vi "Connect To Replacement Terminal.vi"(6 "replacement class term":refnum<vi>, 9 "endpt subvi":refnum<vi>) -> ()   [LabVIEW 2020, in "NI_TargetHelper.lvlib"]
uses:
  <vilib>/TargetSupport/NI_TargetHelper/NI_TargetHelper.lvlib
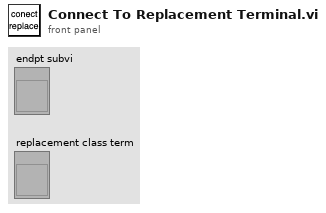
[diagram p1: front panel]
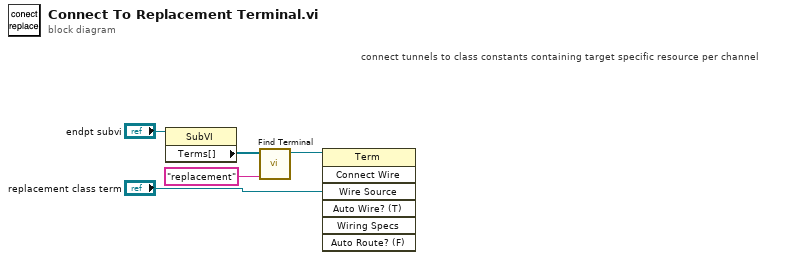
[diagram p0: block diagram]
diagram:
  # "connect tunnels to class constants containing target specific resource per channel"
  n1 = property class="SubVI"(reference="endpt subvi") -> ("Terms[]"=w3:refnum<vi>[])  [unwired: 1 in, 2 out]
  n2 = call <vilib>:"Find Terminal.vi"("terminal name"="replacement" ("y"), "Terminals[]"=w3) -> ("terminal"=w1:refnum<vi>)  [unwired: 9 in]
  n3 = invoke class="Term" method="Connect Wire"(reference=w1, "Wire Source"="replacement class term") -> ()  [unwired: 5 in, 7 out]
